vi "cm_XControlStateFGV.vi"(7 "Action":T1=enum."Write", 10 "Running?":bool, 11 "XControl Name":string) -> (0 "Array 2":bool[](array[boolean]), 1 "Array":string[](array[string]), 2 "Found":bool, 3 "Running?":bool)   [LabVIEW 2012, in "Channel Monitor.xctl"]
uses:
  Channel Monitor.xctl
  cm_XControlState Action.ctl
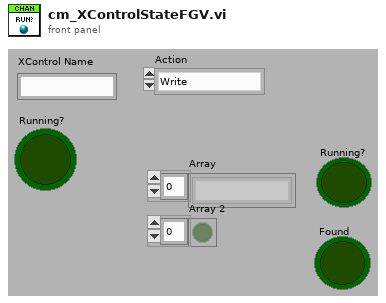
[diagram p1: front panel]
types:
  T1 = typedef "Channel Monitor.xctl/cm_XControlState Action.ctl" = enum16{"Add", "Write", "Read", "Remove"}
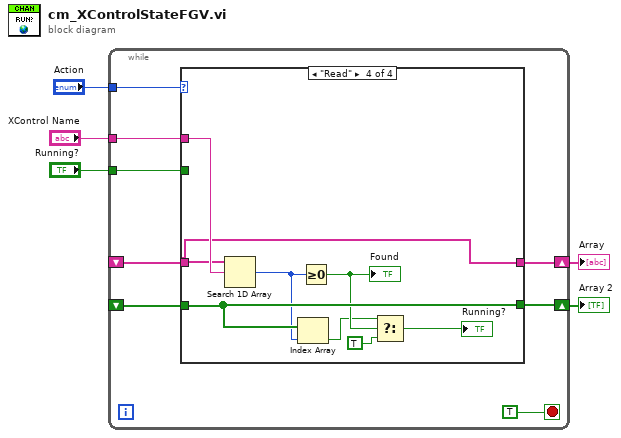
[diagram p0: block diagram]
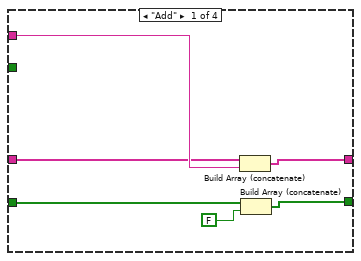
[diagram p2: hidden frame]
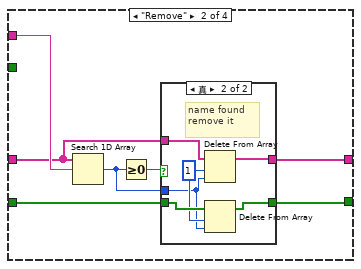
[diagram p3: hidden frame]
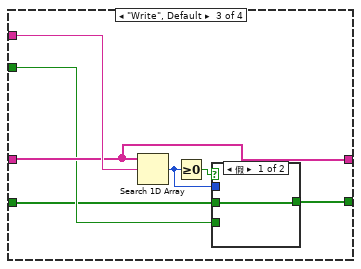
[diagram p5: hidden frame]
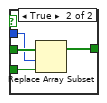
[diagram p6: hidden frame]
diagram:
  n1 = while {
    shift-right: [w9] -> w2
    shift-left: _ -> [w8]
    tunnel: "Action" -> [w12]
    tunnel: "XControl Name" -> [w11]
    tunnel: "Running?" -> [w10]
    shift-right: [w7] -> w1
    shift-left: _ -> [w6]
    stop <- TRUE stop-if-true
    n2 = case shown="\"Read\"" w12 {
      tunnel: w11 -> [w19 w26 w41 w54]
      tunnel: w10 -> [_ _ w39 _]
      tunnel: [w17 w21 w40 w53] -> w9
      tunnel: w8 -> [w18 w24 w40 w53]
      tunnel: [w15 w22 w38 w52] -> w7
      tunnel: w6 -> [w16 w23 w37 w52]
      frame "Add" {
        n3 = Build Array (concatenate)(w18, w19) -> (w17:string[])
        n4 = Build Array (concatenate)(w16, FALSE) -> (w15:bool[])
      }
      frame "Remove" {
        n5 = Search 1D Array(1D array=w24, element=w26) -> (index of element=w20:i32)  [unwired: 1 in]
        n6 = Greater Or Equal To 0?(x=w20) -> (x >= 0?=w25:bool)
        n7 = case shown="真" w25 {
          tunnel: w24 -> [w27 w34]
          tunnel: w23 -> [w28 w32]
          tunnel: [w28 w31] -> w22
          tunnel: [w27 w33] -> w21
          tunnel: w20 -> [_ w29]
          frame False {
            # "not found\ndo nothing"
          }
          frame True {
            w30 = 1 ("length")
            # "name found\nremove it"
            n8 = Delete From Array(array=w34, length=w30, index=w29) -> (array with subset deleted=w33:string[])  [unwired: 1 out]
            n9 = Delete From Array(array=w32, length=w30, index=w29) -> (array with subset deleted=w31:bool[])  [unwired: 1 out]
          }
        }
      }
      frame "Write", Default {
        n10 = Search 1D Array(1D array=w40, element=w41) -> (index of element=w36:i32)  [unwired: 1 in]
        n11 = Greater Or Equal To 0?(x=w36) -> (x >= 0?=w35:bool)
        n12 = case shown="假" w35 {
          tunnel: w39 -> [_ w46]
          tunnel: [w42 w45] -> w38
          tunnel: w37 -> [w42 w44]
          tunnel: w36 -> [_ w43]
          frame False {
          }
          frame True {
            n13 = Replace Array Subset(array=w44, new element=w46, index=w43) -> (w45:bool[])
          }
        }
      }
      frame "Read" {
        n14 = Search 1D Array(1D array=w53, element=w54) -> (index of element=w51:i32)  [unwired: 1 in]
        n15 = Index Array(array=w52, index=w51) -> (element=w49:bool)
        n16 = Greater Or Equal To 0?(x=w51) -> (x >= 0?=w50:bool)
        "Found" <- w50
        n17 = Select(t=w49, s=w50, f=TRUE) -> (s? t:f=→"Running?":bool)
      }
    }
  }
  "Array" <- w2
  "Array 2" <- w1
